vi "ex3-6.vi"() -> ()   [LabVIEW 2009]
panel:
  out "警示燈 >0.75?":bool
  in  "結束":bool
  out "Sine 波形圖":dbl(graph)
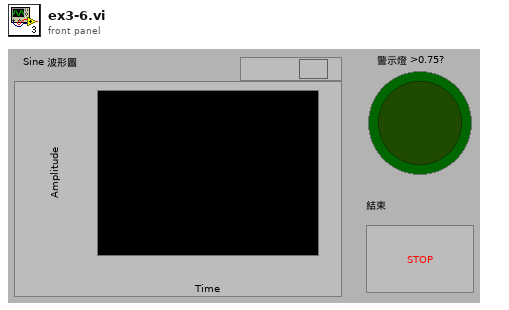
[diagram p1: front panel]
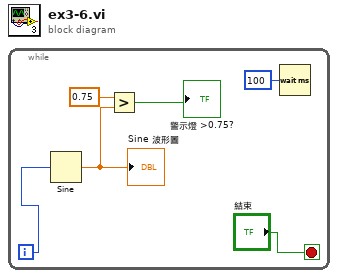
[diagram p0: block diagram]
diagram:
  n1 = while {
    i -> [w6]
    stop <- "結束" stop-if-true
    n2 = Sine(x=w6) -> (sin(x)=w3:dbl)
    "Sine 波形圖" <- w3
    n3 = Greater?(x=0.75, y=w3) -> (0:→"警示燈 >0.75?":bool)
    n4 = Wait (ms)(milliseconds to wait=u32 100) -> ()  [unwired: 1 out]
  }
